vi "Create.vi"(7 "Direction":T1, 8 "error in (no error)":errorcluster, 9 "Custom Config Data":u8[](array[numeric]), 10 "Name":string, 11 "CIFTag in":refnum<class "CIF_NIChn_Fifo_Power_DVR.lvclass">) -> (0 "error out":errorcluster, 3 "CIFTag out":refnum<class "CIF_NIChn_Fifo_Power_DVR.lvclass">)   [LabVIEW 2021, in "CIF_NIChn_Fifo_Power_DVR.lvclass"]
uses:
  CIF_NIChn_Fifo_Power_DVR.lvclass
  CIFChannels/CIFChannels.lvclass
  CIFChannels/Typedef/Disconnect Behavior.ctl
  CIFChannels/Typedef/Channel State.ctl
  05c6e502-0377-480c-a15d-085597602460.vi
  c6f1aac1-fdda-4143-8087-f9e7d57e6170.vi
  ChannelCommon/typedef/Datatype Waveform.ctl
  ChannelCommon/ChannelCommon.lvlib
  D:/dev/CIF-LVCore/src/Channels/CIFChannels/CIFChannels.lvclass
  CIFChannels/Typedef/Direction.ctl
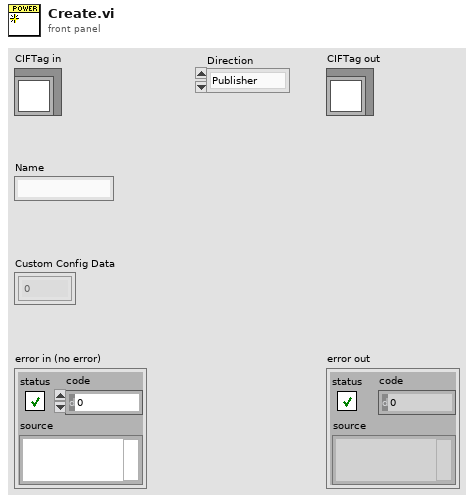
[diagram p1: front panel]
types:
  T1 = typedef "CIFChannels.lvclass/Direction.ctl" = enum16{"Publisher", "Subscriber"}
  T2 = typedef "CIFChannels.lvclass/Disconnect Behavior.ctl" = enum16{"Default value", "Last value", "Error with default"}
  T3 = typedef "ChannelCommon.lvlib/Datatype Waveform.ctl" = cluster{"measurement":dbl[], "dT":dbl, "Timestamp":i64, "Read Lock":bool}
  T4 = typedef "CIFChannels.lvclass/Channel State.ctl" = enum16{"Creating", "Disconnected", "Connecting", "Connected", "Destroyed"}
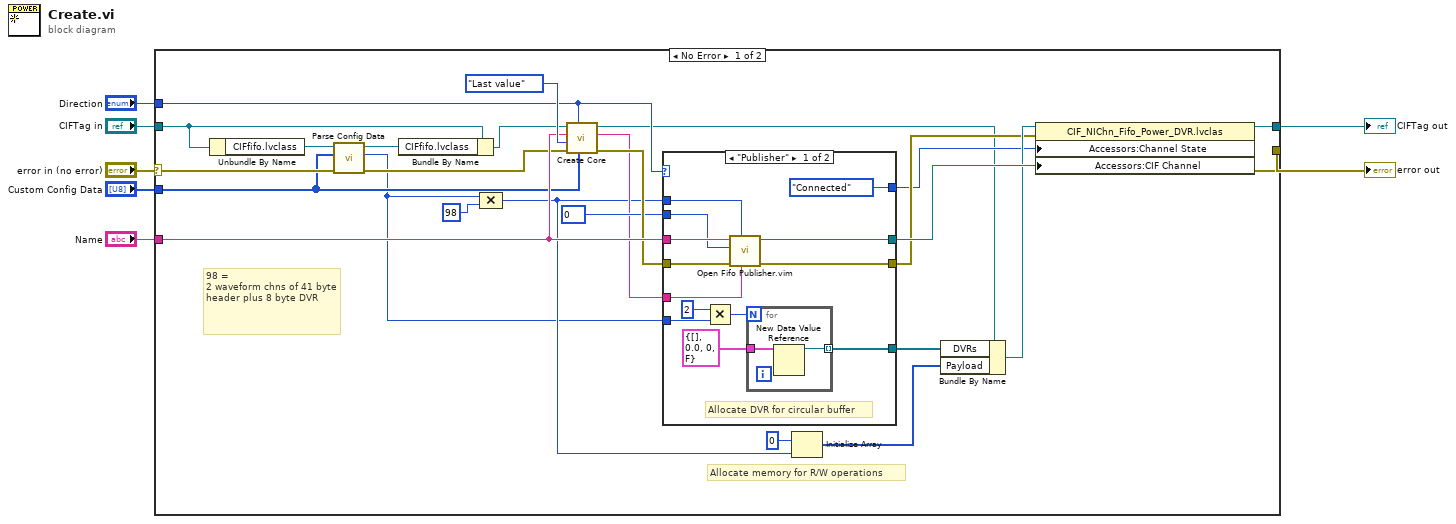
[diagram p0: block diagram]
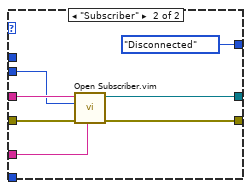
[diagram p2: hidden frame]
diagram:
  n1 = case shown="No Error" "error in (no error)" {
    selector: "error in (no error)" -> [w16 w57]
    tunnel: [w32 w57] -> w6
    tunnel: [w26 w56] -> w4
    tunnel: "CIFTag in" -> [w19 w56]
    tunnel: "Name" -> [w31 _]
    tunnel: "Direction" -> [w25 _]
    tunnel: "Custom Config Data" -> [w14 _]
    frame No Error {
      # "98 =\n2 waveform chns of 41 byte header plus 8 byte DVR"
      # "Allocate memory for R/W operations"
      n2 = Unbundle By Name(w19) -> ("CIFfifo.lvclass"=w18:refnum<class "CIFfifo.lvclass">)
      n3 = call "Parse Config Data.vi"("error in (no error)"=w16, "Custom Config Data"=w14, "CIFfifo in"=w18) -> ("error out"=w15:errorcluster, "Depth"=w9:u64, "CIFfifo out"=w17:refnum<class "CIFfifo.lvclass">)  [unwired: 6 in]
      n4 = Bundle By Name(cluster=w19, "CIFfifo.lvclass"=w17) -> (w21:refnum<class "CIF_NIChn_Fifo_Power_DVR.lvclass">)
      n5 = Compound Arithmetic op=MULTIPLY(w9, u64 98 ("y")) -> (w11:u64)
      n6 = call "Create Core.vi"("Custom Config Data"=w14, "Direction"=w25, "error in (no error)"=w15, "Disconnect Behavior"=Disconnect_Behavior."Last value", "Name"=w31, "CIFChannels in"=w21) -> ("error out"=w30:errorcluster, "Channel Type"=w20:string, "CIFChannels out"=w23:refnum<class "CIF_NIChn_Fifo_Power_DVR.lvclass">)  [unwired: 1 in, 2 out]
      n7 = case shown="\"Publisher\"" w25 {
        tunnel: w31 -> [w46 w54]
        tunnel: w30 -> [w45 w53]
        tunnel: [w41 w49] -> w29
        tunnel: [w42 w50] -> w27
        tunnel: w20 -> [w44 w52]
        tunnel: [Channel_State."Connected" ("Channel State") Channel_State."Disconnected" ("Channel State")] -> w24
        tunnel: u8 0 -> [w40 w51]
        tunnel: w11 -> [w39 _]
        tunnel: w9 -> [w37 _]
        tunnel: [w38 _] -> w8
        frame "Publisher" {
          # "Allocate DVR for circular buffer"
          n8 = Multiply(x=u64 2, y=w37) -> (x*y=w36:u64)
          n9 = call "Open Fifo Publisher.vim"("Channel Type Description"=w44, "depth"=w39, "error in"=w45, "Input Type"=w40, "Channel Name"=w46) -> ("error out"=w42:errorcluster, "CIF Channel"=w41:refnum<k21>)  [unwired: 5 in]
          n10 = for {
            N: w36 -> [_]
            tunnel: T3 {"measurement"=[], "dT"=0.0, "Timestamp"=0, "Read Lock"=FALSE} ("Waveform Datatype") -> [w48]
            tunnel: [w47] -> w38 mode=indexing
            n11 = New Data Value Reference(data value=w48) -> (data value reference=w47:refnum<data-value>)  [unwired: 1 in, 1 out]
          }
        }
        frame "Subscriber" {
          n12 = call "Open Subscriber.vim"("Channel Type Description"=w52, "error in"=w53, "Input Type"=w51, "Channel Name"=w54) -> ("error out"=w50:errorcluster, "CIF Channel"=w49:refnum<k21>)  [unwired: 6 in]
        }
      }
      n13 = Initialize Array(u8 0 ("Numeric"), w11) -> (w10:u8[])
      n14 = Bundle By Name(cluster=w23, "DVRs"=w8, "Payload"=w10) -> (w28:refnum<class "CIF_NIChn_Fifo_Power_DVR.lvclass">)
      n15 = property class="CIF_NIChn_Fifo_Power_DVR.lvclas"(reference=w28, error in=w27, "Accessors:Channel State"=w24, "Accessors:CIF Channel"=w29) -> (reference out=w26:refnum<class "CIF_NIChn_Fifo_Power_DVR.lvclass">, error out=w32:errorcluster)
    }
    frame Error {
    }
  }
  "error out" <- w6
  "CIFTag out" <- w4
